vi "WaveGeneratorSub.vi"(4 "TestLoops":i32, 5 "Data array":dbl[](array[numeric]), 6 "dt":dbl, 7 "Wave":T1 items=["0指令", "正弦波", "方波", "三角波", "常值", "波形数据", "白噪声", "正弦扫频", "梯度加载", "VMIC"], 8 "deltaF":dbl, 9 "Offset":dbl, 10 "Frequent":dbl, 11 "Amplitude":dbl) -> (3 "Output":dbl)   [LabVIEW 2014]
uses:
  WaveType.ctl
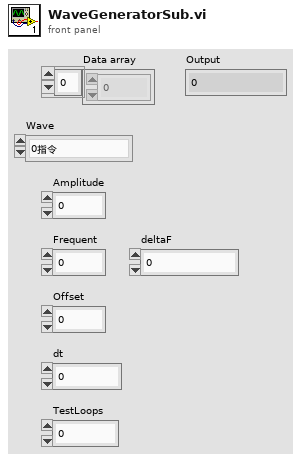
[diagram p1: front panel]
types:
  T1 = typedef "WaveType.ctl" = i32
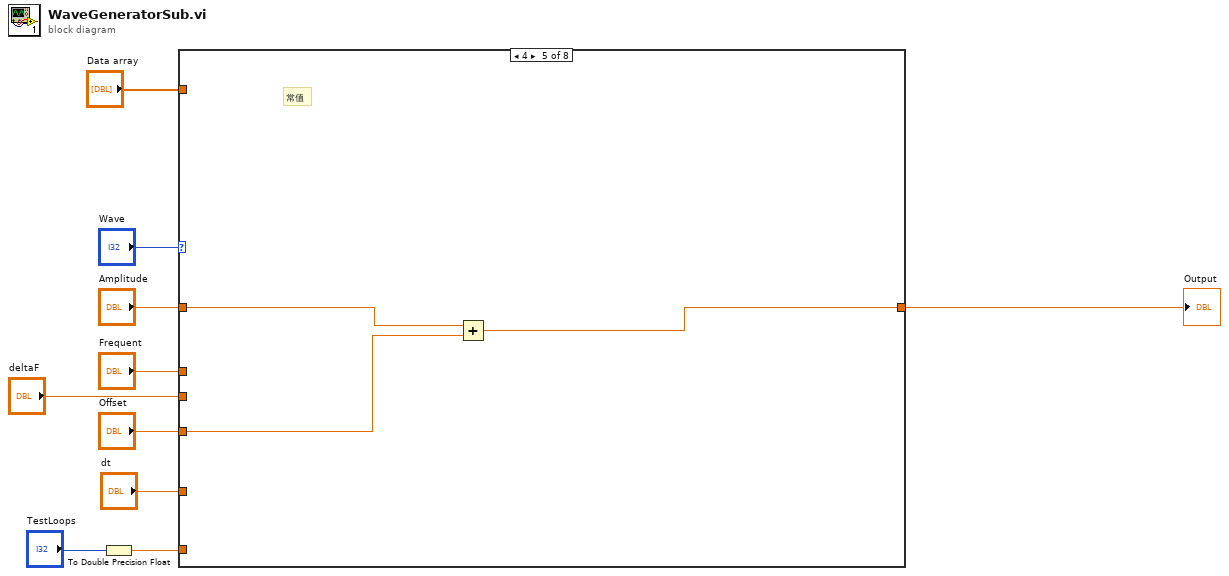
[diagram p0: block diagram]
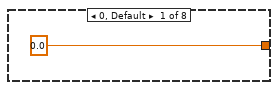
[diagram p2: hidden frame]
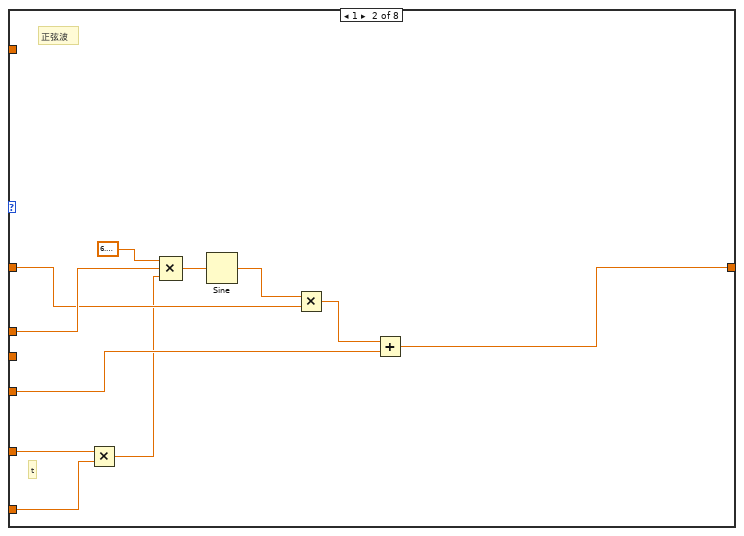
[diagram p3: hidden frame]
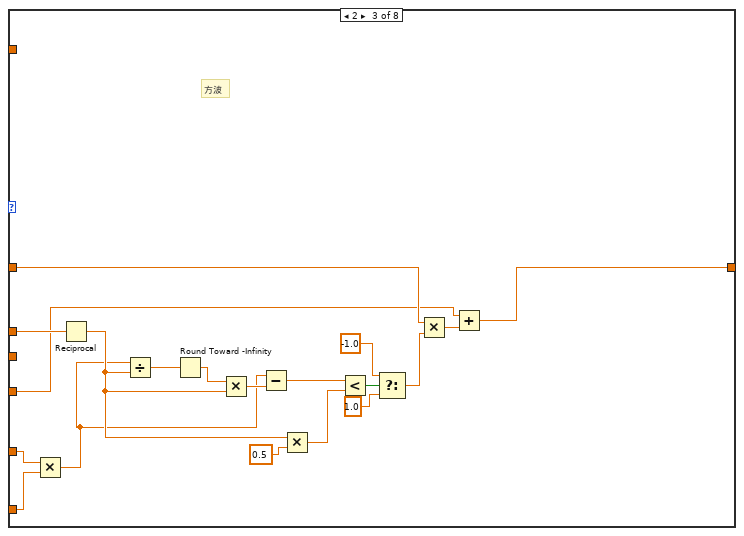
[diagram p4: hidden frame]
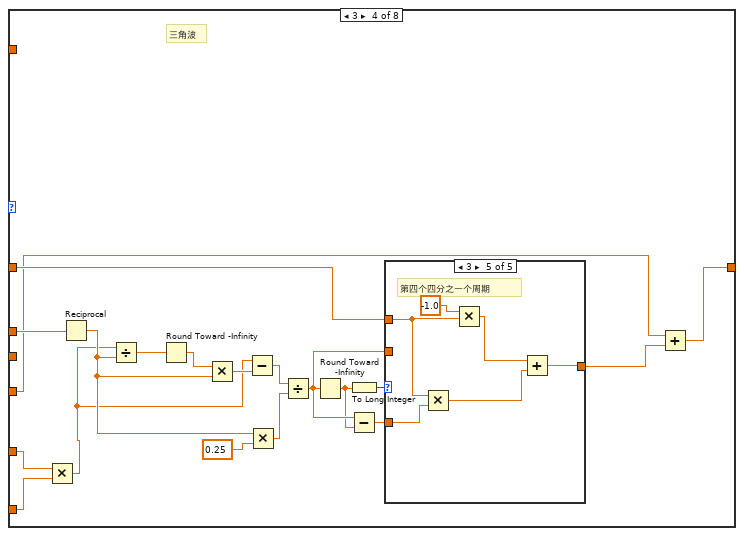
[diagram p5: hidden frame]
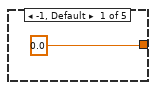
[diagram p6: hidden frame]
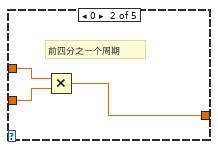
[diagram p7: hidden frame]
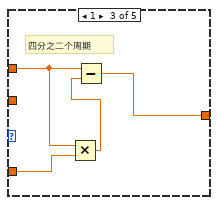
[diagram p8: hidden frame]
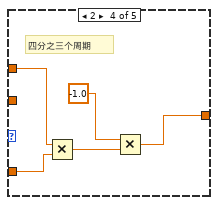
[diagram p9: hidden frame]
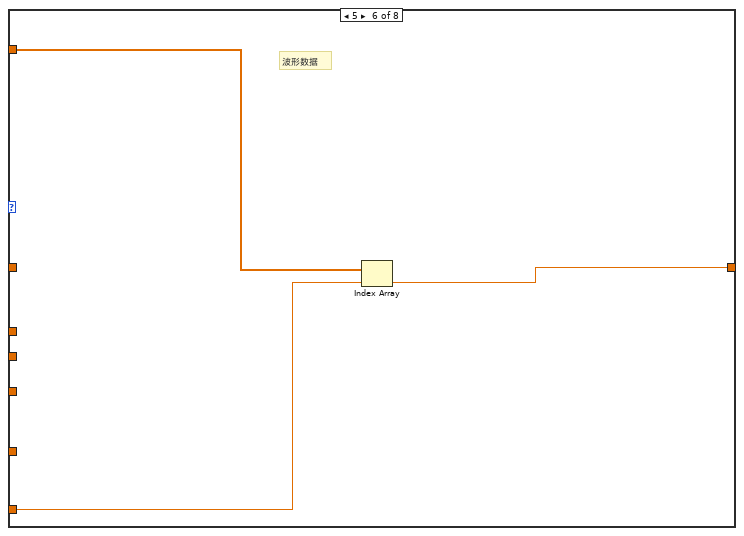
[diagram p10: hidden frame]
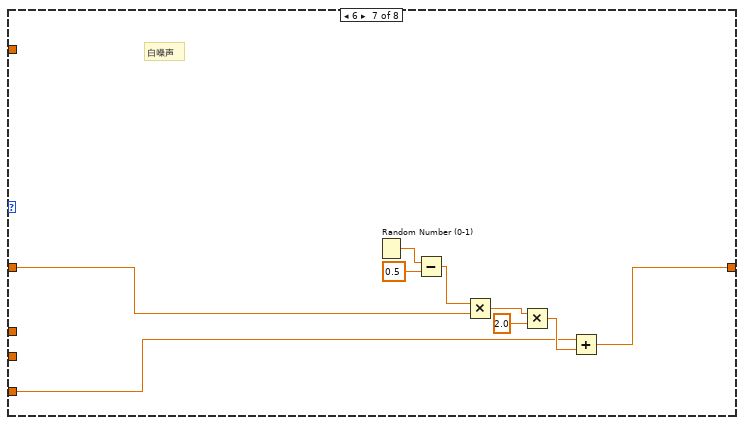
[diagram p11: hidden frame]
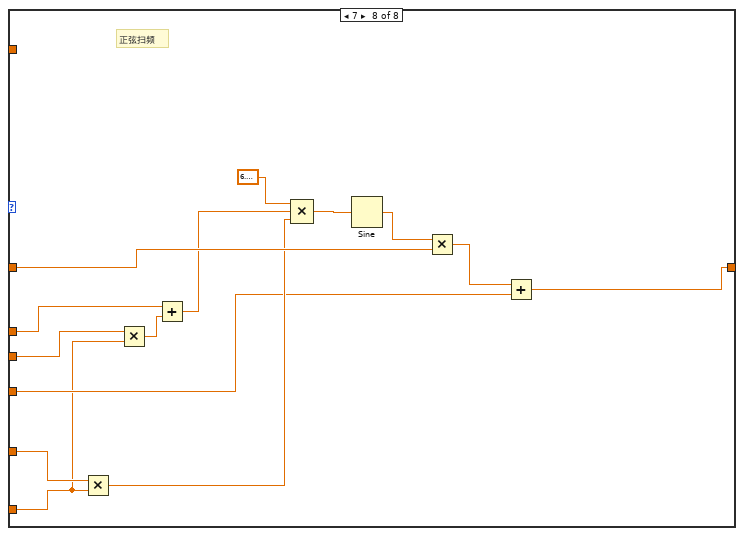
[diagram p12: hidden frame]
diagram:
  n1 = To Double Precision Float(number="TestLoops") -> (double precision float=w2:dbl)
  n2 = case shown="4" "Wave" {
    tunnel: "dt" -> [_ w16 w25 w44 _ _ _ w102]
    tunnel: "Amplitude" -> [_ w19 w29 w52 w81 _ w94 w103]
    tunnel: "Frequent" -> [_ w21 w41 w60 _ _ _ w96]
    tunnel: "Offset" -> [_ w17 w27 w46 w82 _ w87 w100]
    tunnel: [0.0 w14 w26 w45 w80 w83 w86 w104] -> w3
    tunnel: "Data array" -> [_ _ _ _ _ w85 _ _]
    tunnel: w2 -> [_ w12 w24 w43 _ w84 _ w98]
    tunnel: "deltaF" -> [_ _ _ _ _ _ _ w99]
    frame 0, Default {
    }
    frame 1 {
      # "t"
      # "正弦波"
      n3 = Multiply(x=w16, y=w12) -> (x*y=w13:dbl)
      n4 = Compound Arithmetic op=MULTIPLY(6.283185307179586, w21, w13) -> (w15:dbl)
      n5 = Sine(x=w15) -> (sin(x)=w20:dbl)
      n6 = Multiply(x=w20, y=w19) -> (x*y=w18:dbl)
      n7 = Add(x=w18, y=w17) -> (x+y=w14:dbl)
    }
    frame 2 {
      # "方波"
      n8 = Multiply(x=w25, y=w24) -> (x*y=w23:dbl)
      n9 = Reciprocal(x=w41) -> (1/x=w36:dbl)
      n10 = Divide(x=w23, y=w36) -> (x/y=w40:dbl)
      n11 = Round Toward -Infinity(1:w40) -> (0:w39:dbl)
      n12 = Multiply(x=w39, y=w36) -> (x*y=w38:dbl)
      n13 = Subtract(x=w23, y=w38) -> (x-y=w37:dbl)
      n14 = Multiply(x=w36, y=0.5) -> (x*y=w34:dbl)
      n15 = Less?(x=w37, y=w34) -> (x < y?=w33:bool)
      n16 = Select(t=-1.0, s=w33, f=1.0) -> (s? t:f=w30:dbl)
      n17 = Multiply(x=w29, y=w30) -> (x*y=w28:dbl)
      n18 = Add(x=w27, y=w28) -> (x+y=w26:dbl)
    }
    frame 3 {
      # "三角波"
      n19 = Multiply(x=w44, y=w43) -> (x*y=w42:dbl)
      n20 = Reciprocal(x=w60) -> (1/x=w55:dbl)
      n21 = Divide(x=w42, y=w55) -> (x/y=w59:dbl)
      n22 = Round Toward -Infinity(1:w59) -> (0:w58:dbl)
      n23 = Multiply(x=w58, y=w55) -> (x*y=w57:dbl)
      n24 = Subtract(x=w42, y=w57) -> (x-y=w51:dbl)
      n25 = Multiply(x=w55, y=0.25) -> (x*y=w54:dbl)
      n26 = Divide(x=w51, y=w54) -> (x/y=w50:dbl)
      n27 = Round Toward -Infinity(1:w50) -> (0:w49:dbl)
      n28 = To Long Integer(number=w49) -> (32bit integer=w53:i32)
      n29 = Subtract(x=w50, y=w49) -> (x-y=w48:dbl)
      n30 = case shown="3" w53 {
        tunnel: w52 -> [_ w64 w65 w72 w76]
        tunnel: [0.0 w62 w66 w69 w77] -> w47
        tunnel: w50 -> [_ w63 _ _ _]
        tunnel: w48 -> [_ _ w68 w73 w79]
        frame -1, Default {
        }
        frame 0 {
          # "前四分之一个周期"
          n31 = Multiply(x=w64, y=w63) -> (x*y=w62:dbl)
        }
        frame 1 {
          # "四分之二个周期"
          n32 = Multiply(x=w65, y=w68) -> (x*y=w67:dbl)
          n33 = Subtract(x=w65, y=w67) -> (x-y=w66:dbl)
        }
        frame 2 {
          # "四分之三个周期"
          n34 = Multiply(x=w72, y=w73) -> (x*y=w71:dbl)
          n35 = Multiply(x=-1.0, y=w71) -> (x*y=w69:dbl)
        }
        frame 3 {
          # "第四个四分之一个周期"
          n36 = Multiply(x=w76, y=w79) -> (x*y=w75:dbl)
          n37 = Multiply(x=-1.0, y=w76) -> (x*y=w74:dbl)
          n38 = Add(x=w74, y=w75) -> (x+y=w77:dbl)
        }
      }
      n39 = Add(x=w46, y=w47) -> (x+y=w45:dbl)
    }
    frame 4 {
      # "常值"
      n40 = Add(x=w81, y=w82) -> (x+y=w80:dbl)
    }
    frame 5 {
      # "波形数据"
      n41 = Index Array(array=w85, index=w84) -> (element=w83:dbl)
    }
    frame 6 {
      # "白噪声"
      n42 = Random Number (0-1)() -> (number: 0 to 1=w93:dbl)
      n43 = Subtract(x=w93, y=0.5) -> (x-y=w91:dbl)
      n44 = Multiply(x=w91, y=w94) -> (x*y=w90:dbl)
      n45 = Multiply(x=w90, y=2.0) -> (x*y=w88:dbl)
      n46 = Add(x=w87, y=w88) -> (x+y=w86:dbl)
    }
    frame 7 {
      # "正弦扫频"
      n47 = Multiply(x=w102, y=w98) -> (x*y=w101:dbl)
      n48 = Multiply(x=w99, y=w98) -> (x*y=w97:dbl)
      n49 = Add(x=w96, y=w97) -> (x+y=w95:dbl)
      n50 = Compound Arithmetic op=MULTIPLY(6.283185307179586, w95, w101) -> (w105:dbl)
      n51 = Sine(x=w105) -> (sin(x)=w107:dbl)
      n52 = Multiply(x=w107, y=w103) -> (x*y=w106:dbl)
      n53 = Add(x=w106, y=w100) -> (x+y=w104:dbl)
    }
  }
  "Output" <- w3
